vi "ForLoopExample_Fibonacci.vi"() -> ()   [LabVIEW 2020]
panel:
  out "Ciag Fibonacciego wykres":i32[](graph)
  out "Ciag Fibonacciego, n=19":i32[](array[numeric])
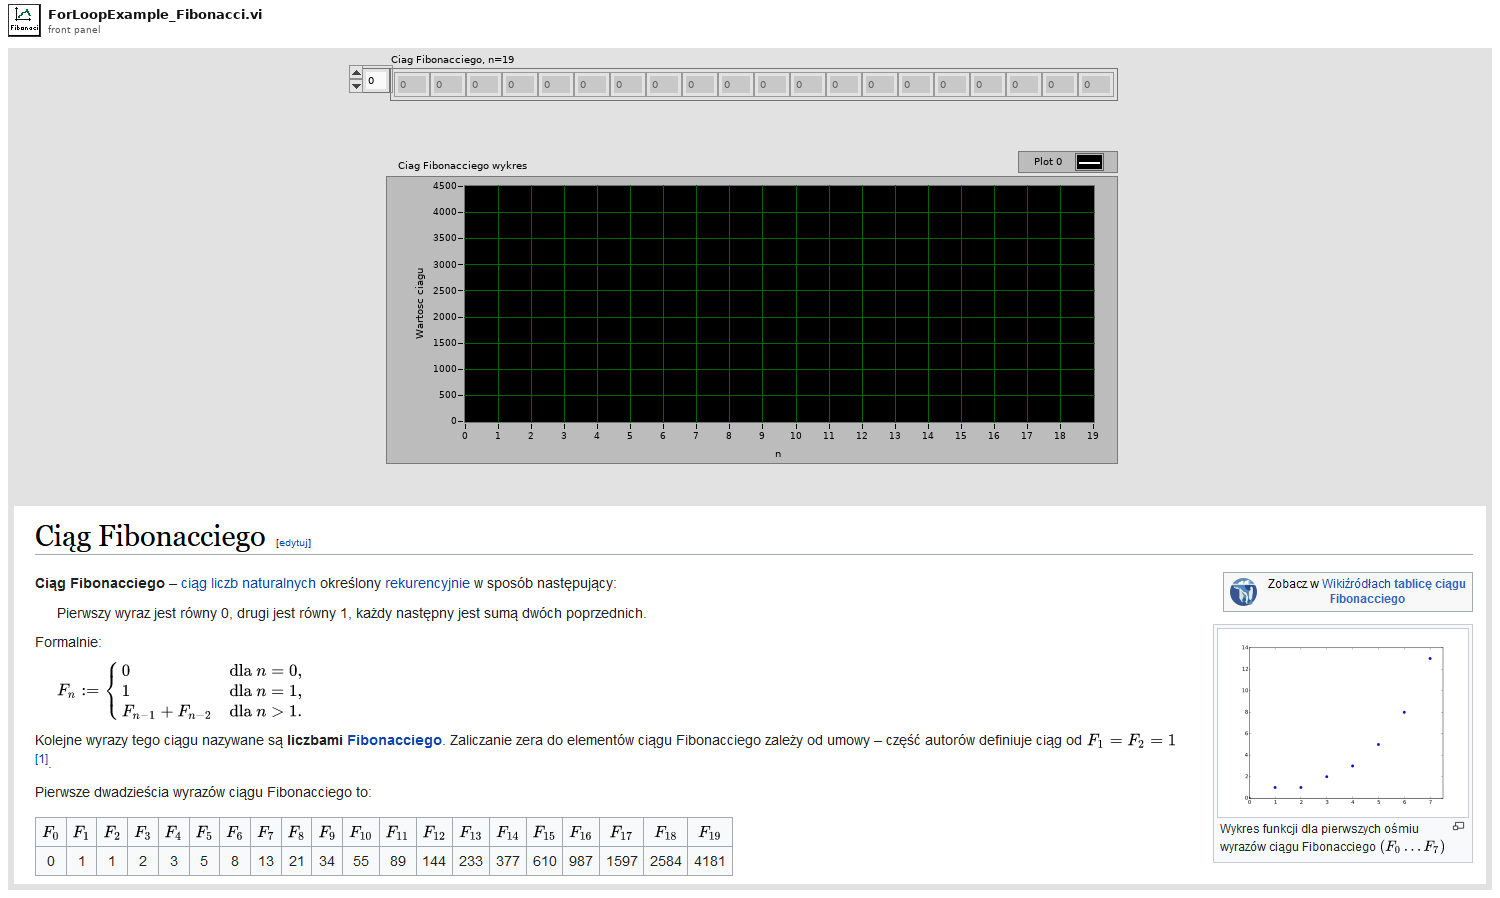
[diagram p1: front panel]
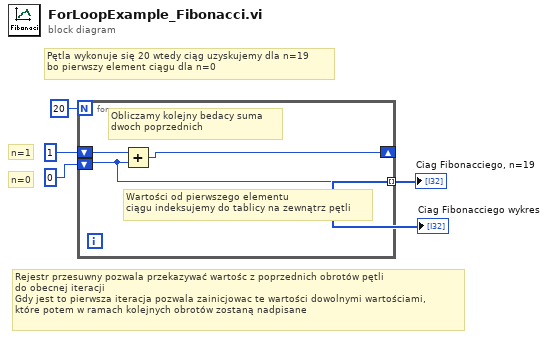
[diagram p0: block diagram]
diagram:
  # "Rejestr przesuwny pozwala przekazywać wartośc z poprzednich obrotów pętli\ndo obecnej iteracji \nGdy jest to pierwsza iteracja pozwala zainicjowac te wartości dowolnymi wartościami,\nktóre potem w ramach kolejnych obrotów zostaną nadpisane"
  # "n=1"
  # "n=0"
  # "Pętla wykonuje się 20 wtedy ciąg uzyskujemy dla n=19\nbo pierwszy element ciągu dla n=0"
  n1 = for {
    N: 20 -> [_]
    shift-right: [w6] -> _
    shift-left: 1 -> [w7]
    shift-left: 0 -> [w5]
    tunnel: [w5] -> w1 mode=indexing
    # "Wartości od pierwszego elementu\nciągu indeksujemy do tablicy na zewnątrz pętli"
    # "Obliczamy kolejny bedacy suma\ndwoch poprzednich"
    n2 = Add(x=w7, y=w5) -> (x+y=w6:i32)
  }
  "Ciag Fibonacciego, n=19" <- w1
  "Ciag Fibonacciego wykres" <- w1
